vi "thermo_get_reading.vi"(7 "force read":bool, 8 "error in":errorcluster, 11 "thermo":T2={"type"=enum."COMET Tx5xx (ethernet)", "comment"="", "tag"="", "refresh"=5.0, "IP"="192.168.2.34", "port"=502, "VISA"="", "last readout"=timestamp(0 s since 1904-01-01), "TCP ref"=refnum, "VISA sess"="", "idn"="", "press"=0.0, "RH"=0.0, "temp"=0.0, "pres cor"=[], "RH cor"=[], "temp cor"=[], "try left"=0, "failed"=FALSE, "RTD set"=[], "RTD inv"=[], "range"=0.0, "net mode"=enum."MODBUS", "try fail"=enum."Stop trying - return NaN", "timeout [s]"=0.0, "max retries"=0, "sim t [deg]"=0.0} {"RTD inv" format="%.1f"; "RTD set" format="%.1f"; "temp cor" format="%.1f"; "RH cor" format="%.1f"; "pres cor" format="%.1f"; "refresh" min=0.1 max=1000.0 format="%.2f"}) -> (0 "error out":errorcluster, 1 "RH [%]":dbl, 2 "temp [deg C]":dbl, 3 "thermo out":T2={"type"=enum."COMET Tx5xx (ethernet)", "comment"="", "tag"="", "refresh"=5.0, "IP"="192.168.2.34", "port"=502, "VISA"="", "last readout"=timestamp(0 s since 1904-01-01), "TCP ref"=refnum, "VISA sess"="", "idn"="", "press"=0.0, "RH"=0.0, "temp"=0.0, "pres cor"=[], "RH cor"=[], "temp cor"=[], "try left"=0, "failed"=FALSE, "RTD set"=[], "RTD inv"=[], "range"=0.0, "net mode"=enum."MODBUS", "try fail"=enum."Stop trying - return NaN", "timeout [s]"=0.0, "max retries"=0, "sim t [deg]"=0.0} {"RTD inv" format="%.1f"; "RTD set" format="%.1f"; "temp cor" format="%.1f"; "RH cor" format="%.1f"; "pres cor" format="%.1f"; "refresh" min=0.1 max=1000.0 format="%.2f"}, 4 "p [Pa]":dbl, 5 "reading":T1, 6 "status code":i32)   [LabVIEW 2020]
uses:
  thermo.ctl
  thermo_types.ctl
  Thermometer Fail Action.ctl
  thermo_read.ctl
  thermo_var.vi
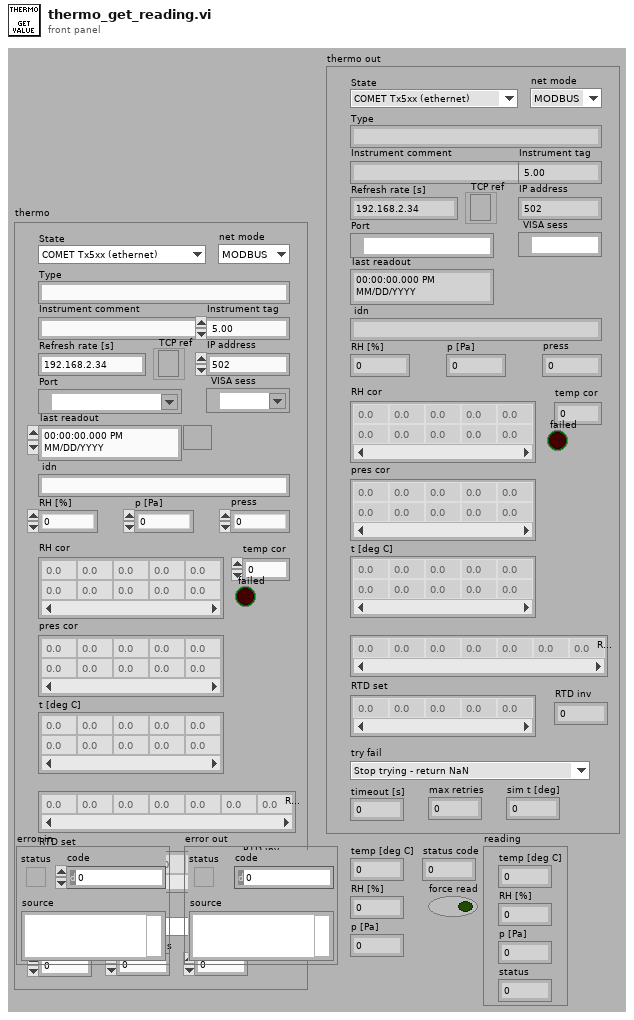
[diagram p1: front panel]
types:
  T1 = typedef "thermo_read.ctl" = cluster{"temp [deg C]":dbl, "RH [%]":dbl, "p [Pa]":dbl, "status":i32}
  T2 = typedef "thermo.ctl" = cluster{"type":T3, "comment":string, "tag":string, "refresh":dbl, "IP":string, "port":u16, "VISA":refnum<visa-resource-name>, "last readout":timestamp, "TCP ref":refnum<k5>, "VISA sess":refnum<visa-resource-name>, "idn":string, "press":dbl, "RH":dbl, "temp":dbl, "pres cor":dbl[][], "RH cor":dbl[][], "temp cor":dbl[][], "try left":i32, "failed":bool, "RTD set":dbl[], "RTD inv":dbl[], "range":dbl, "net mode":enum16{"MODBUS", "HTTP"}, "try fail":T4, "timeout [s]":dbl, "max retries":i32, "sim t [deg]":dbl}
  T3 = typedef "thermo_types.ctl" = enum16{"Disabled", "Simulated", "COMET Tx5xx (ethernet)", "Keithley 2002 (GPIB) + RTD", "Agilent 344xx (GPIB) + RTD"}
  T4 = typedef "Thermometer Fail Action.ctl" = enum16{"Stop trying - keep last value", "Stop trying - return NaN", "Generate error - stop sweep"}
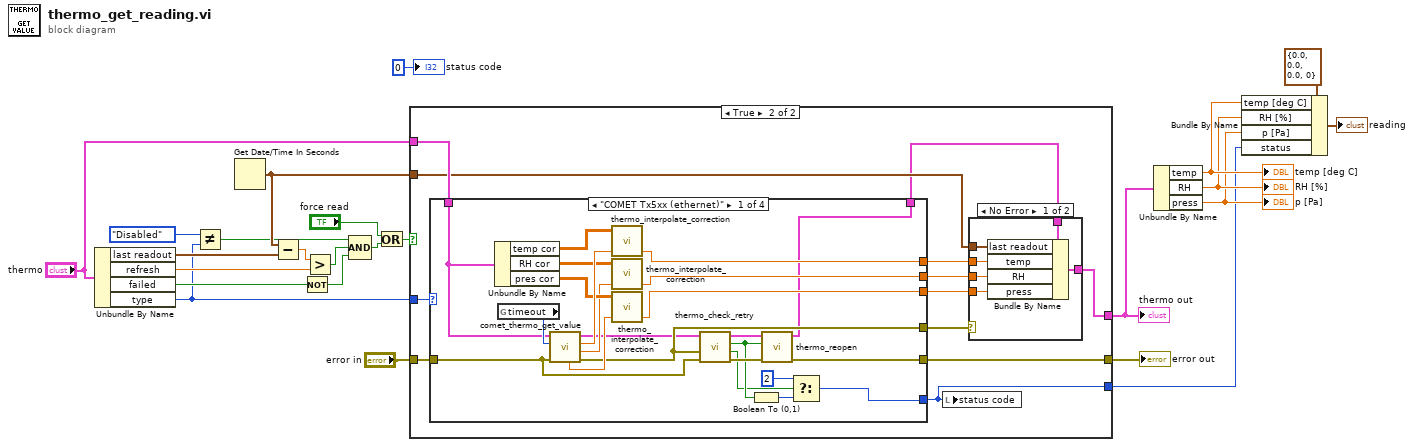
[diagram p0: block diagram]
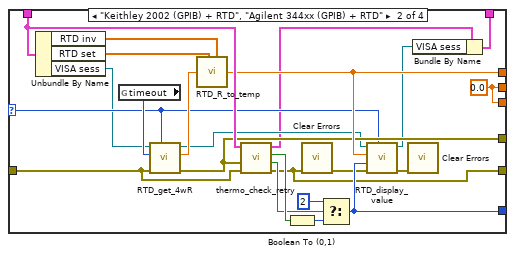
[diagram p4: hidden frame]
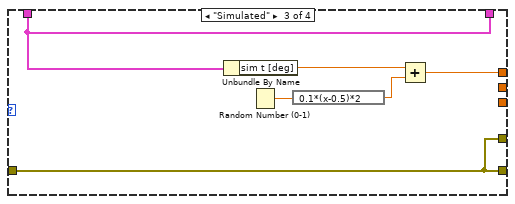
[diagram p5: hidden frame]
diagram:
  n1 = Unbundle By Name("thermo") -> ("last readout"=w18:timestamp, "refresh"=w23:dbl, "failed"=w13:bool, "type"=w9:T3)
  n2 = Not Equal?(x=thermo_types."Disabled", y=w9) -> (x != y?=w8:bool)
  n3 = Get Date/Time In Seconds() -> (seconds since 1Jan1904=w19:timestamp)
  n4 = Subtract(x=w19, y=w18) -> (x-y=w24:dbl)
  n5 = Not(x=w13) -> (.not. x?=w12:bool)
  n6 = Greater?(x=w24, y=w23) -> (0:w22:bool)
  n7 = Compound Arithmetic op=AND(w8, w22, w12) -> (w16:bool)
  n8 = Or(x="force read", y=w16) -> (x .or. y?=w17:bool)
  n9 = case shown="True" w17 {
    tunnel: w9 -> [_ w38]
    tunnel: "error in" -> [w26 w37]
    tunnel: [w26 w36] -> w10
    tunnel: "thermo" -> [w25 w35]
    tunnel: w19 -> [_ w31]
    tunnel: [w25 w28] -> w14
    tunnel: [_ w27] -> w2
    frame False {
    }
    frame True {
      n10 = case shown="\"COMET Tx5xx (ethernet)\"" w38 {
        selector: w38 -> [_ w77 _ _]
        tunnel: [w56 w76 w97 w99] -> w36
        tunnel: w37 -> [w59 w89 w97 w99]
        tunnel: [w66 w81 w92 _] -> w34
        tunnel: [w65 w88 _ _] -> w33
        tunnel: [w63 w88 _ _] -> w32
        tunnel: w35 -> [w48 w87 w96 w98]
        tunnel: [w58 w80 w97 w99] -> w30
        tunnel: [w50 w78 _ _] -> w27
        tunnel: [w46 w69 w96 w98] -> w29
        frame "COMET Tx5xx (ethernet)" {
          n11 = Unbundle By Name(w48) -> ("temp cor"=w68:dbl[][], "RH cor"=w64:dbl[][], "pres cor"=w62:dbl[][])
          n12 = global read "thermo_var.vi" "timeout"() -> (w49:i32)
          n13 = call "comet_thermo_get_value.vi"("error in"=w59, "timeout (5000)"=w49, "thermo in"=w48) -> ("error out"=w58:errorcluster, "RH [%]"=w61:dbl, "t [C]"=w67:dbl, "thermo out"=w47:T2, "p [hPa]"=w60:dbl)  [unwired: 3 in, 1 out]
          n14 = call "thermo_interpolate_correction.vi"("input"=w67, "temp cor"=w68) -> ("output"=w66:dbl)  [unwired: 1 in, 2 out]
          n15 = call "thermo_interpolate_correction.vi"("input"=w61, "temp cor"=w64) -> ("output"=w65:dbl)  [unwired: 1 in, 2 out]
          n16 = call "thermo_interpolate_correction.vi"("input"=w60, "temp cor"=w62) -> ("output"=w63:dbl)  [unwired: 1 in, 2 out]
          n17 = call "thermo_check_retry.vi"("error in"=w59, "thermo error in"=w58, "thermo in"=w47) -> ("error out"=w57:errorcluster, "fail"=w53:bool, "retry"=w54:bool, "thermo out"=w55:T2)  [unwired: 5 in]
          n18 = Boolean To (0,1)(Boolean=w54) -> (0, 1=w52:i16)
          n19 = call "thermo_reopen.vi"("error in"=w57, "allow reopen"=w54, "thermo in"=w55) -> ("error out"=w56:errorcluster, "thermo out"=w46:T2)  [unwired: 6 in, 1 out]
          n20 = Select(t=i16 2, s=w53, f=w52) -> (s? t:f=w50:i16)
        }
        frame "Keithley 2002 (GPIB) + RTD", "Agilent 344xx (GPIB) + RTD" {
          w88 = 0.0 ("output")
          n21 = Unbundle By Name(w87) -> ("RTD inv"=w73:dbl[], "RTD set"=w86:dbl[], "VISA sess"=w72:refnum<visa-resource-name>)
          n22 = global read "thermo_var.vi" "timeout"() -> (w84:i32)
          n23 = call "RTD_get_4wR.vi"("type"=w77, "error in"=w89, "timeout [ms]"=w84, "VISA in"=w72) -> ("error out"=w80:errorcluster, "R value [Ohm]"=w85:dbl, "VISA out"=w79:refnum<visa-resource-name>)  [unwired: 5 in]
          n24 = call "RTD_R_to_temp.vi"("RTD coefficients"=w86, "R [Ohm]"=w85, "RTD inverse poly"=w73) -> ("t [deg C]"=w81:dbl)  [unwired: 6 in]
          n25 = call "thermo_check_retry.vi"("error in"=w89, "thermo error in"=w80, "thermo in"=w87) -> ("error out"=w76:errorcluster, "fail"=w90:bool, "retry"=w91:bool, "thermo out"=w70:T2)  [unwired: 5 in]
          n26 = Boolean To (0,1)(Boolean=w91) -> (0, 1=w82:i16)
          n27 = call <vilib>:"Clear Errors.vi"("error in (no error)"=w76) -> ("error out"=w75:errorcluster)  [unwired: 5 in, 1 out]
          n28 = Select(t=i16 2, s=w90, f=w82) -> (s? t:f=w78:i16)
          n29 = call "RTD_display_value.vi"("type"=w77, "error in"=w75, "status code"=w78, "temp [deg C]"=w81, "VISA in"=w79) -> ("error out"=w74:errorcluster, "VISA out"=w71:refnum<visa-resource-name>)  [unwired: 5 in]
          n30 = call <vilib>:"Clear Errors.vi"("error in (no error)"=w74) -> ()  [unwired: 5 in, 2 out]
          n31 = Bundle By Name(cluster=w70, "VISA sess"=w71) -> (w69:T2)
        }
        frame "Simulated" {
          n32 = Unbundle By Name(w96) -> ("sim t [deg]"=w93:dbl)
          n33 = Random Number (0-1)() -> (number: 0 to 1=w95:dbl)
          n34 = expression code="0.1*(x-0.5)*2"(w95) -> (w94:dbl)
          n35 = Add(x=w93, y=w94) -> (x+y=w92:dbl)
        }
        frame Default {
        }
      }
      n36 = local write "status code"(w27) -> ()
      n37 = case shown="No Error" w30 {
        tunnel: [w44 w45] -> w28
        tunnel: w29 -> [w43 w45]
        tunnel: w34 -> [w42 _]
        tunnel: w33 -> [w41 _]
        tunnel: w32 -> [w40 _]
        tunnel: w31 -> [w39 _]
        frame No Error {
          n38 = Bundle By Name(cluster=w43, "last readout"=w39, "temp"=w42, "RH"=w41, "press"=w40) -> (w44:T2)
        }
        frame Error {
        }
      }
    }
  }
  "error out" <- w10
  "thermo out" <- w14
  n39 = Unbundle By Name(w14) -> ("temp"=w5:dbl, "RH"=w4:dbl, "press"=w3:dbl)
  "temp [deg C]" <- w5
  "RH [%]" <- w4
  "p [Pa]" <- w3
  n40 = Bundle By Name(cluster=T1 {"temp [deg C]"=0.0, "RH [%]"=0.0, "p [Pa]"=0.0, "status"=0} ("thermo"), "temp [deg C]"=w5, "RH [%]"=w4, "p [Pa]"=w3, "status"=w2) -> (→"reading":T1)
  "status code" <- 0 ("status code")
